vi "FpgaLink_Open.vi"(8 "error in (no error)":errorcluster, 11 "VP":string) -> (0 "error out":errorcluster, 2 "VP Out":string, 3 "handle out":i64)   [LabVIEW 2011]
doc: "Open a connection to the FPGALink device at the specified VID & PID.\n\nConnects to the device and verifies it is an FPGALink device, then queries its capabilities and synchronises the USB bulk endpoints."
uses:
  <vilib>/Utility/importsl/GetValueByPointer/datatype.ctl
  <vilib>/Utility/importsl/GetValueByPointer/GetValueByPointer.xnode
  resource/lvimptsl.dll
  libfpgalink.dll
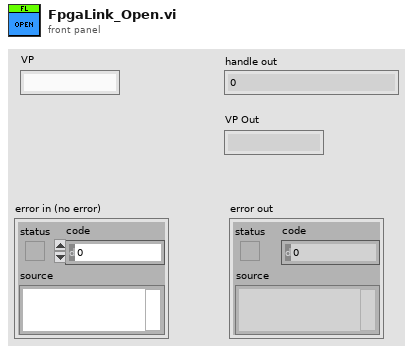
[diagram p1: front panel]
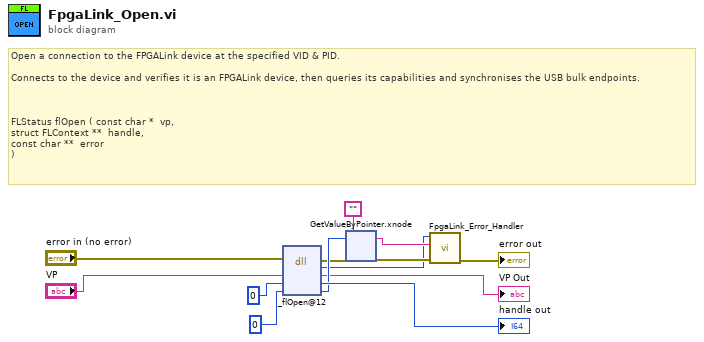
[diagram p0: block diagram]
diagram:
  # "Open a connection to the FPGALink device at the specified VID & PID.\n\nConnects to the device and verifies it is an FPGALink device, then queries its capabilities and synchronises the USB bulk endpoints.\n\n\n\nFLStatus flOpen\t(\tconst char * \tvp,\nstruct FLContext ** \thandle,\nconst char ** \terror \n)"
  n1 = dll-call lib="libfpgalink.*" fn="_flOpen@12"(error in="error in (no error)", "vp"="VP", "handle"=i64 0, "error"=i64 0 ("error_out")) -> (error out=w9:errorcluster, "FLStatus"=w3:u32, "vp"=→"VP Out":string, "handle"=→"handle out":i64, "error"=w10:i64)  [unwired: 2 in, 1 out]
  n2 = xnode "GetValueByPointer.xnode"("Pointer"=w10, "InputType"="", "ErrorIn"=w9) -> ("Output"=w6:string, "ErrorOut"=w7:errorcluster)  [unwired: 1 in]
  n3 = call <vilib>:"FpgaLink_Error_Handler.vi"("error in (no error)"=w7, "error string"=w6, "error code"=w3) -> ("error out"=→"error out":errorcluster)  [unwired: 8 in]
